vi "temp chart with pid BAP5B.vi"(1 "exit T control":bool, 7 "Control Parameters":T4={"Setpoint"=50.0, "Control bandwidth"=4.0, "Settle bandwidth"=1.0, "Integral time"=30.0, "Int\non"=TRUE, "Derivative time"=0.5, "Der\non"=TRUE, "Settle time"=60.0} {"Settle time" format="%.2f"; "Derivative time" format="%.2f"; "Integral time" format="%.2f"; "Settle bandwidth" format="%.2f"; "Control bandwidth" format="%.2f"; "Setpoint" format="%.2f"}, 11 "error in":errorcluster) -> (8 "Temp":dbl format="%.2f", 15 "error out":errorcluster)   [LabVIEW 2014]
doc: "temp chart with power BAP5B\n\nIn run time records, plots, and displays how the temperature of a \"bug,\" an assortment of a capacitor, thermistor, and resistor is affected by normalized power. This uses ELVIS II multimeter as the measuring device. \n\nBeverly Abadines\nPHY 350"
uses:
  typedefs/control parameters.ctl
panel:
  in  "Manual Override":bool
  in  "Scale Control":T1
  in  "Power Control":dbl(slide) scale=0.0..1.0
  out "range indicators":T2={"In control band"=FALSE, "In settle band"=FALSE, "under range"=TRUE, "over range"=FALSE}
  out "Power":dbl=0.754407202908737 format="%.2f"
  out "Setpoint":dbl=50.0 format="%.2f"
  out "Temperature History":T3(graph)={"temp out"=29.702811899974034, 50.0, 50.5, 49.5, 50.1, 49.9, 50.508814405817475}
  # "Automatic Temperature Controller"
  # "1.0"
  # "Norm\nPower\nscale"
  # "0.5"
  # "0.0"
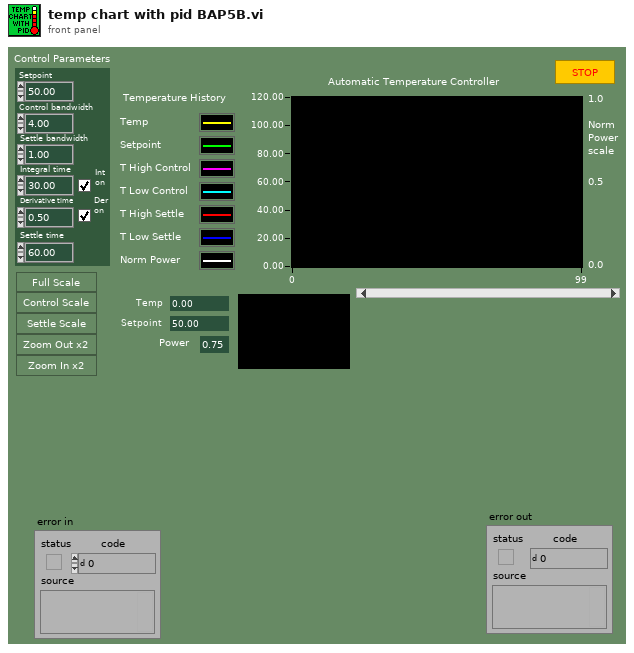
[diagram p1: front panel]
types:
  T1 = cluster{"Full Scale":bool, "Control Scale":bool, "Settle Scale":bool, "Zoom Out":bool, "Zoom In":bool}
  T2 = cluster{"In control band":bool, "In settle band":bool, "under range":bool, "over range":bool}
  T3 = cluster{"temp out":dbl, dbl, dbl, dbl, dbl, dbl, dbl}
  T4 = typedef "control parameters.ctl" = cluster{"Setpoint":dbl, "Control bandwidth":dbl, "Settle bandwidth":dbl, "Integral time":dbl, "Int\non":bool, "Derivative time":dbl, "Der\non":bool, "Settle time":dbl}
  T5 = cluster{"[0]":refnum<vi>, "[1]":refnum<vi>, "[2]":refnum<vi>, "[3]":refnum<vi>}
  T6 = typedef "status indicator.ctl" = cluster{"In control band":bool, "In settle band":bool, "under range":bool, "over range":bool}
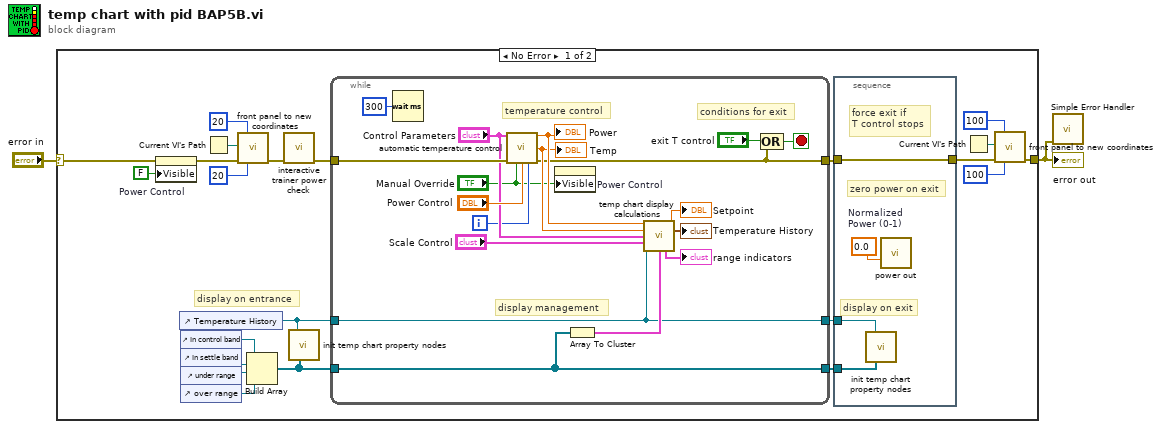
[diagram p0: block diagram]
diagram:
  n1 = case shown="No Error" "error in" {
    selector: "error in" -> [w5 w47]
    tunnel: [w9 w47] -> w1
    frame No Error {
      # "display on entrance"
      n2 = property on="Power Control" class="Slide (strict)"(error in=w5, "Visible"=FALSE) -> (error out=w3:errorcluster)  [unwired: 1 in, 1 out]
      n3 = control-ref of="Temperature History"() -> (w22:refnum<vi>)
      n4 = control-ref of="In control band"() -> (w16:refnum<vi>)
      n5 = control-ref of="In settle band"() -> (w17:refnum<vi>)
      n6 = control-ref of="under range"() -> (w18:refnum<vi>)
      n7 = control-ref of="over range"() -> (w19:refnum<vi>)
      n8 = Current VI's Path() -> (path=w13:path)
      n9 = call "front panel to new coordinates.vi"("new top"=i16 20, "path"=w13, "error in (no error)"=w3, "new left"=i16 20) -> ("error out"=w7:errorcluster)  [unwired: 11 in]
      n10 = Build Array(w16, w17, w18, w19) -> (w23:refnum<vi>[])
      n11 = call "interactive trainer power check.vi"("error in"=w7) -> ("error out"=w6:errorcluster)  [unwired: 14 in]
      n12 = call "init temp chart property nodes.vi"("Temperature History"=w22, "range indicators"=w23) -> ()  [unwired: 4 in, 10 out]
      n13 = while {
        tunnel: [w32] -> w20
        tunnel: [w33] -> w21
        tunnel: w22 -> [w32]
        tunnel: w23 -> [w33]
        tunnel: w6 -> [w35]
        tunnel: [w28] -> w24
        i -> [w26]
        stop <- w36 stop-if-true
        # "display management"
        # "conditions for exit"
        # "temperature control"
        n14 = Wait (ms)(milliseconds to wait=u32 300) -> ()  [unwired: 1 out]
        n15 = call "automatic temperature control.vi"("Control Parameters"="Control Parameters", "error in"=w35, "Manual Override"="Manual Override", "Normalized Power In (0-1)"="Power Control", "index (0=init)"=w26) -> ("power meas (0-1)"=w31:dbl, "temp meas"=w30:dbl, "error out"=w28:errorcluster)  [unwired: 6 in, 2 out]
        "Temp" <- w30
        "Power" <- w31
        n16 = property on="Power Control" class="Slide (strict)"("Visible"="Manual Override") -> ()  [unwired: 2 in, 2 out]
        n17 = Array To Cluster(array=w33) -> (cluster=w34:T5)
        n18 = call "temp chart display calculations.vi"("power in (0-1)"=w31, "temp in"=w30, "Control Parameters"="Control Parameters", "Scale Control In"="Scale Control", "Temp History in"=w32, "range indicator refs"=w34) -> ("Setpoint out"=→"Setpoint":dbl, "Temperature History out"=→"Temperature History":T3, "range indicators out"=→"range indicators":T6)  [unwired: 3 in, 4 out]
        n19 = Compound Arithmetic op=OR("exit T control", w28) -> (w36:bool)
      }
      n20 = stacked-sequence {
        tunnel: [w46] -> w8
        tunnel: w24 -> [w46]
        tunnel: w21 -> [w44]
        tunnel: w20 -> [w43]
        frame #0 {
          w45 = 0.0  # Normalized Power (0-1)
          # "display on exit"
          # "force exit if \nT control stops"
          # "zero power on exit"
          n21 = call "init temp chart property nodes.vi"("Temperature History"=w43, "range indicators"=w44) -> ()  [unwired: 4 in, 10 out]
          n22 = call "power out.vi"("Normalized Power (0-1)"=w45) -> ()  [unwired: 2 in, 13 out]
        }
      }
      n23 = Current VI's Path() -> (path=w10:path)
      n24 = call "front panel to new coordinates.vi"("new top"=i16 100, "path"=w10, "error in (no error)"=w8, "new left"=i16 100) -> ("error out"=w9:errorcluster)  [unwired: 11 in]
    }
    frame Error {
    }
  }
  "error out" <- w1
  n25 = call <vilib>:"Simple Error Handler.vi"("error in (no error)"=w1) -> ()  [unwired: 4 in, 5 out]
